vi "Lab Panel V5.20.vi"() -> ()   [LabVIEW 2013] (continued)
                      tunnel: w3938 -> [_ w3961]
                      frame #0 {
                        n2199 = case shown="True" w3955 {
                          tunnel: w3954 -> [_ w3960]
                          tunnel: w3953 -> [_ w3959]
                          tunnel: w3952 -> [_ w3958]
                          tunnel: w3951 -> [_ w3956]
                          frame False {
                          }
                          frame True {
                            n2200 = Bundle(cluster=w3956, "amps"=w3960, "volts"=w3959, "pf"=w3958) -> (w3957:cluster{"amps":dbl, "volts":dbl, "pf":dbl})
                            n2201 = local write "ON L01-2"(w3957) -> ()
                          }
                        }
                      }
                      frame #1 {
                        n2202 = Unbundle(w3965) -> ("amps"=w3964:dbl, "volts"=w3963:dbl, "pf"=w3962:dbl)
                        n2203 = case shown="True" w3966 {
                          tunnel: w3973 -> [_ w4005]
                          tunnel: w3972 -> [_ w4012]
                          tunnel: w3971 -> [_ _]
                          tunnel: w3970 -> [_ _]
                          tunnel: w3969 -> [_ w4011]
                          tunnel: w3968 -> [_ w4010]
                          tunnel: w3967 -> [_ w3975]
                          tunnel: w3964 -> [_ w4007]
                          tunnel: w3963 -> [_ w4006]
                          tunnel: w3962 -> [_ w4004]
                          tunnel: w3961 -> [_ w3996]
                          frame False {
                          }
                          frame True {
                            n2204 = local read "TDMS LAB01-2"() -> (w4009:refnum<k34>)
                            n2205 = Build Array(w4006) -> (w4001:dbl[])
                            n2206 = Build Array(w4004) -> (w4000:dbl[])
                            n2207 = Build Array(w4011) -> (w3999:dbl[])
                            n2208 = Build Array(w4012) -> (w3998:dbl[])
                            n2209 = Build Array(w4007) -> (w4003:dbl[])
                            n2210 = Build Array(w4005) -> (w4002:dbl[])
                            n2211 = Build Array(w4010) -> (w3997:dbl[])
                            n2212 = Build Array("AMPS ON", "AMPS OFF", "VOLTS", "PF", "TEMP Live", "TEMP Neut", "CYCLE") -> (w3980:string[])
                            n2213 = Bundle By Name("Y"=w4003, "t0"=w3996) -> (w3995:waveform(dbl))  [unwired: 1 in]
                            n2214 = Bundle By Name("Y"=w4002, "t0"=w3996) -> (w3994:waveform(dbl))  [unwired: 1 in]
                            n2215 = Bundle By Name("Y"=w4001, "t0"=w3996) -> (w3993:waveform(dbl))  [unwired: 1 in]
                            n2216 = Bundle By Name("Y"=w4000, "t0"=w3996) -> (w3992:waveform(dbl))  [unwired: 1 in]
                            n2217 = Bundle By Name("Y"=w3999, "t0"=w3996) -> (w3991:waveform(dbl))  [unwired: 1 in]
                            n2218 = Bundle By Name("Y"=w3998, "t0"=w3996) -> (w3990:waveform(dbl))  [unwired: 1 in]
                            n2219 = Bundle By Name("Y"=w3997, "t0"=w3996) -> (w3989:waveform(dbl))  [unwired: 1 in]
                            n2220 = Build Array(w3995, w3994, w3993, w3992, w3991, w3990, w3989) -> (w3988:waveform(dbl)[])
                            n2221 = TDMS Write(0:w4009, 5:"TEST VALUES", 7:w3980, 9:w3988) -> (4:w3979:refnum<k34>, 6:w3978:string, 15:w3977:errorcluster)  [unwired: 2 in, 1 out]
                            n2222 = TDMS Write(0:w3979, 5:w3978, 7:"TIME", 9:w3975, 11:w3977) -> (15:w3974:errorcluster)  [unwired: 1 in, 3 out]
                            n2223 = local write "data file error"(w3974) -> ()
                          }
                        }
                      }
                    }
                  }
                }
              }
              frame #2 {
                n2224 = case shown="True" w4013 {
                  tunnel: w4017 -> [_ w4022]
                  tunnel: w4016 -> [_ w4021]
                  tunnel: w4015 -> [_ w4019]
                  tunnel: w4014 -> [_ w4018]
                  frame False {
                  }
                  frame True {
                    n2225 = local read "DISP LAB02-1"() -> (w4023:T4)
                    n2226 = local read "SIG LAB02-1"() -> (w4024:T2)
                    n2227 = local read "ON L02-1"() -> (w4020:cluster{"amps":dbl, "volts":dbl, "pf":dbl})
                    n2228 = Unbundle(w4024) -> ("AMPS"=w4030:dbl, "VOLTS"=w4028:dbl, "PF"=w4027:dbl, "Tmp Live"=w4026:dbl, "Tmp Neut"=w4029:dbl)
                    n2229 = Unbundle(w4023) -> ("CYCLE"=w4025:dbl)  [unwired: 2 out]
                    n2230 = stacked-sequence {
                      tunnel: w4030 -> [w4034 w4053]
                      tunnel: w4029 -> [_ w4052]
                      tunnel: w4028 -> [w4033 w4051]
                      tunnel: w4027 -> [w4032 w4050]
                      tunnel: w4026 -> [_ w4049]
                      tunnel: w4025 -> [_ w4048]
                      tunnel: w4022 -> [_ w4047]
                      tunnel: w4021 -> [w4035 _]
                      tunnel: w4020 -> [w4031 w4045]
                      tunnel: w4019 -> [_ w4046]
                      tunnel: w4018 -> [_ w4041]
                      frame #0 {
                        n2231 = case shown="True" w4035 {
                          tunnel: w4034 -> [_ w4040]
                          tunnel: w4033 -> [_ w4039]
                          tunnel: w4032 -> [_ w4038]
                          tunnel: w4031 -> [_ w4036]
                          frame False {
                          }
                          frame True {
                            n2232 = Bundle(cluster=w4036, "amps"=w4040, "volts"=w4039, "pf"=w4038) -> (w4037:cluster{"amps":dbl, "volts":dbl, "pf":dbl})
                            n2233 = local write "ON L02-1"(w4037) -> ()
                          }
                        }
                      }
                      frame #1 {
                        n2234 = Unbundle(w4045) -> ("amps"=w4044:dbl, "volts"=w4043:dbl, "pf"=w4042:dbl)
                        n2235 = case shown="True" w4046 {
                          tunnel: w4053 -> [_ w4085]
                          tunnel: w4052 -> [_ w4092]
                          tunnel: w4051 -> [_ _]
                          tunnel: w4050 -> [_ _]
                          tunnel: w4049 -> [_ w4091]
                          tunnel: w4048 -> [_ w4090]
                          tunnel: w4047 -> [_ w4055]
                          tunnel: w4044 -> [_ w4087]
                          tunnel: w4043 -> [_ w4086]
                          tunnel: w4042 -> [_ w4084]
                          tunnel: w4041 -> [_ w4076]
                          frame False {
                          }
                          frame True {
                            n2236 = local read "TDMS LAB02-1"() -> (w4089:refnum<k34>)
                            n2237 = Build Array(w4086) -> (w4081:dbl[])
                            n2238 = Build Array(w4084) -> (w4080:dbl[])
                            n2239 = Build Array(w4091) -> (w4079:dbl[])
                            n2240 = Build Array(w4092) -> (w4078:dbl[])
                            n2241 = Build Array(w4087) -> (w4083:dbl[])
                            n2242 = Build Array(w4085) -> (w4082:dbl[])
                            n2243 = Build Array(w4090) -> (w4077:dbl[])
                            n2244 = Build Array("AMPS ON", "AMPS OFF", "VOLTS", "PF", "TEMP Live", "TEMP Neut", "CYCLE") -> (w4060:string[])
                            n2245 = Bundle By Name("Y"=w4083, "t0"=w4076) -> (w4075:waveform(dbl))  [unwired: 1 in]
                            n2246 = Bundle By Name("Y"=w4082, "t0"=w4076) -> (w4074:waveform(dbl))  [unwired: 1 in]
                            n2247 = Bundle By Name("Y"=w4081, "t0"=w4076) -> (w4073:waveform(dbl))  [unwired: 1 in]
                            n2248 = Bundle By Name("Y"=w4080, "t0"=w4076) -> (w4072:waveform(dbl))  [unwired: 1 in]
                            n2249 = Bundle By Name("Y"=w4079, "t0"=w4076) -> (w4071:waveform(dbl))  [unwired: 1 in]
                            n2250 = Bundle By Name("Y"=w4078, "t0"=w4076) -> (w4070:waveform(dbl))  [unwired: 1 in]
                            n2251 = Bundle By Name("Y"=w4077, "t0"=w4076) -> (w4069:waveform(dbl))  [unwired: 1 in]
                            n2252 = Build Array(w4075, w4074, w4073, w4072, w4071, w4070, w4069) -> (w4068:waveform(dbl)[])
                            n2253 = TDMS Write(0:w4089, 5:"TEST VALUES", 7:w4060, 9:w4068) -> (4:w4059:refnum<k34>, 6:w4058:string, 15:w4057:errorcluster)  [unwired: 2 in, 1 out]
                            n2254 = TDMS Write(0:w4059, 5:w4058, 7:"TIME", 9:w4055, 11:w4057) -> (15:w4054:errorcluster)  [unwired: 1 in, 3 out]
                            n2255 = local write "data file error"(w4054) -> ()
                          }
                        }
                      }
                    }
                  }
                }
              }
              frame #3 {
                n2256 = case shown="True" w4093 {
                  tunnel: w4097 -> [_ w4102]
                  tunnel: w4096 -> [_ w4101]
                  tunnel: w4095 -> [_ w4099]
                  tunnel: w4094 -> [_ w4098]
                  frame False {
                  }
                  frame True {
                    n2257 = local read "DISP LAB02-2"() -> (w4103:T4)
                    n2258 = local read "SIG LAB02-2"() -> (w4104:T2)
                    n2259 = local read "ON L02-2"() -> (w4100:cluster{"amps":dbl, "volts":dbl, "pf":dbl})
                    n2260 = Unbundle(w4104) -> ("AMPS"=w4110:dbl, "VOLTS"=w4108:dbl, "PF"=w4107:dbl, "Tmp Live"=w4106:dbl, "Tmp Neut"=w4109:dbl)
                    n2261 = Unbundle(w4103) -> ("CYCLE"=w4105:dbl)  [unwired: 2 out]
                    n2262 = stacked-sequence {
                      tunnel: w4110 -> [w4114 w4133]
                      tunnel: w4109 -> [_ w4132]
                      tunnel: w4108 -> [w4113 w4131]
                      tunnel: w4107 -> [w4112 w4130]
                      tunnel: w4106 -> [_ w4129]
                      tunnel: w4105 -> [_ w4128]
                      tunnel: w4102 -> [_ w4127]
                      tunnel: w4101 -> [w4115 _]
                      tunnel: w4100 -> [w4111 w4125]
                      tunnel: w4099 -> [_ w4126]
                      tunnel: w4098 -> [_ w4121]
                      frame #0 {
                        n2263 = case shown="True" w4115 {
                          tunnel: w4114 -> [_ w4120]
                          tunnel: w4113 -> [_ w4119]
                          tunnel: w4112 -> [_ w4118]
                          tunnel: w4111 -> [_ w4116]
                          frame False {
                          }
                          frame True {
                            n2264 = Bundle(cluster=w4116, "amps"=w4120, "volts"=w4119, "pf"=w4118) -> (w4117:cluster{"amps":dbl, "volts":dbl, "pf":dbl})
                            n2265 = local write "ON L02-2"(w4117) -> ()
                          }
                        }
                      }
                      frame #1 {
                        n2266 = Unbundle(w4125) -> ("amps"=w4124:dbl, "volts"=w4123:dbl, "pf"=w4122:dbl)
                        n2267 = case shown="True" w4126 {
                          tunnel: w4133 -> [_ w4165]
                          tunnel: w4132 -> [_ w4172]
                          tunnel: w4131 -> [_ _]
                          tunnel: w4130 -> [_ _]
                          tunnel: w4129 -> [_ w4171]
                          tunnel: w4128 -> [_ w4170]
                          tunnel: w4127 -> [_ w4135]
                          tunnel: w4124 -> [_ w4167]
                          tunnel: w4123 -> [_ w4166]
                          tunnel: w4122 -> [_ w4164]
                          tunnel: w4121 -> [_ w4156]
                          frame False {
                          }
                          frame True {
                            n2268 = local read "TDMS LAB02-2"() -> (w4169:refnum<k34>)
                            n2269 = Build Array(w4166) -> (w4161:dbl[])
                            n2270 = Build Array(w4164) -> (w4160:dbl[])
                            n2271 = Build Array(w4171) -> (w4159:dbl[])
                            n2272 = Build Array(w4172) -> (w4158:dbl[])
                            n2273 = Build Array(w4167) -> (w4163:dbl[])
                            n2274 = Build Array(w4165) -> (w4162:dbl[])
                            n2275 = Build Array(w4170) -> (w4157:dbl[])
                            n2276 = Build Array("AMPS ON", "AMPS OFF", "VOLTS", "PF", "TEMP Live", "TEMP Neut", "CYCLE") -> (w4140:string[])
                            n2277 = Bundle By Name("Y"=w4163, "t0"=w4156) -> (w4155:waveform(dbl))  [unwired: 1 in]
                            n2278 = Bundle By Name("Y"=w4162, "t0"=w4156) -> (w4154:waveform(dbl))  [unwired: 1 in]
                            n2279 = Bundle By Name("Y"=w4161, "t0"=w4156) -> (w4153:waveform(dbl))  [unwired: 1 in]
                            n2280 = Bundle By Name("Y"=w4160, "t0"=w4156) -> (w4152:waveform(dbl))  [unwired: 1 in]
                            n2281 = Bundle By Name("Y"=w4159, "t0"=w4156) -> (w4151:waveform(dbl))  [unwired: 1 in]
                            n2282 = Bundle By Name("Y"=w4158, "t0"=w4156) -> (w4150:waveform(dbl))  [unwired: 1 in]
                            n2283 = Bundle By Name("Y"=w4157, "t0"=w4156) -> (w4149:waveform(dbl))  [unwired: 1 in]
                            n2284 = Build Array(w4155, w4154, w4153, w4152, w4151, w4150, w4149) -> (w4148:waveform(dbl)[])
                            n2285 = TDMS Write(0:w4169, 5:"TEST VALUES", 7:w4140, 9:w4148) -> (4:w4139:refnum<k34>, 6:w4138:string, 15:w4137:errorcluster)  [unwired: 2 in, 1 out]
                            n2286 = TDMS Write(0:w4139, 5:w4138, 7:"TIME", 9:w4135, 11:w4137) -> (15:w4134:errorcluster)  [unwired: 1 in, 3 out]
                            n2287 = local write "data file error"(w4134) -> ()
                          }
                        }
                      }
                    }
                  }
                }
              }
              frame #4 {
                n2288 = case shown="True" w4173 {
                  tunnel: w4177 -> [_ w4182]
                  tunnel: w4176 -> [_ w4181]
                  tunnel: w4175 -> [_ w4179]
                  tunnel: w4174 -> [_ w4178]
                  frame False {
                  }
                  frame True {
                    n2289 = local read "DISP LAB03-1"() -> (w4183:T4)
                    n2290 = local read "SIG LAB03-1"() -> (w4184:T2)
                    n2291 = local read "ON L03-1"() -> (w4180:cluster{"amps":dbl, "volts":dbl, "pf":dbl})
                    n2292 = Unbundle(w4184) -> ("AMPS"=w4190:dbl, "VOLTS"=w4188:dbl, "PF"=w4187:dbl, "Tmp Live"=w4186:dbl, "Tmp Neut"=w4189:dbl)
                    n2293 = Unbundle(w4183) -> ("CYCLE"=w4185:dbl)  [unwired: 2 out]
                    n2294 = stacked-sequence {
                      tunnel: w4190 -> [w4194 w4213]
                      tunnel: w4189 -> [_ w4212]
                      tunnel: w4188 -> [w4193 w4211]
                      tunnel: w4187 -> [w4192 w4210]
                      tunnel: w4186 -> [_ w4209]
                      tunnel: w4185 -> [_ w4208]
                      tunnel: w4182 -> [_ w4207]
                      tunnel: w4181 -> [w4195 _]
                      tunnel: w4180 -> [w4191 w4205]
                      tunnel: w4179 -> [_ w4206]
                      tunnel: w4178 -> [_ w4201]
                      frame #0 {
                        n2295 = case shown="True" w4195 {
                          tunnel: w4194 -> [_ w4200]
                          tunnel: w4193 -> [_ w4199]
                          tunnel: w4192 -> [_ w4198]
                          tunnel: w4191 -> [_ w4196]
                          frame False {
                          }
                          frame True {
                            n2296 = Bundle(cluster=w4196, "amps"=w4200, "volts"=w4199, "pf"=w4198) -> (w4197:cluster{"amps":dbl, "volts":dbl, "pf":dbl})
                            n2297 = local write "ON L03-1"(w4197) -> ()
                          }
                        }
                      }
                      frame #1 {
                        n2298 = Unbundle(w4205) -> ("amps"=w4204:dbl, "volts"=w4203:dbl, "pf"=w4202:dbl)
                        n2299 = case shown="True" w4206 {
                          tunnel: w4213 -> [_ w4245]
                          tunnel: w4212 -> [_ w4252]
                          tunnel: w4211 -> [_ _]
                          tunnel: w4210 -> [_ _]
                          tunnel: w4209 -> [_ w4251]
                          tunnel: w4208 -> [_ w4250]
                          tunnel: w4207 -> [_ w4215]
                          tunnel: w4204 -> [_ w4247]
                          tunnel: w4203 -> [_ w4246]
                          tunnel: w4202 -> [_ w4244]
                          tunnel: w4201 -> [_ w4236]
                          frame False {
                          }
                          frame True {
                            n2300 = local read "TDMS LAB03-1"() -> (w4249:refnum<k34>)
                            n2301 = Build Array(w4246) -> (w4241:dbl[])
                            n2302 = Build Array(w4244) -> (w4240:dbl[])
                            n2303 = Build Array(w4251) -> (w4239:dbl[])
                            n2304 = Build Array(w4252) -> (w4238:dbl[])
                            n2305 = Build Array(w4247) -> (w4243:dbl[])
                            n2306 = Build Array(w4245) -> (w4242:dbl[])
                            n2307 = Build Array(w4250) -> (w4237:dbl[])
                            n2308 = Build Array("AMPS ON", "AMPS OFF", "VOLTS", "PF", "TEMP Live", "TEMP Neut", "CYCLE") -> (w4220:string[])
                            n2309 = Bundle By Name("Y"=w4243, "t0"=w4236) -> (w4235:waveform(dbl))  [unwired: 1 in]
                            n2310 = Bundle By Name("Y"=w4242, "t0"=w4236) -> (w4234:waveform(dbl))  [unwired: 1 in]
                            n2311 = Bundle By Name("Y"=w4241, "t0"=w4236) -> (w4233:waveform(dbl))  [unwired: 1 in]
                            n2312 = Bundle By Name("Y"=w4240, "t0"=w4236) -> (w4232:waveform(dbl))  [unwired: 1 in]
                            n2313 = Bundle By Name("Y"=w4239, "t0"=w4236) -> (w4231:waveform(dbl))  [unwired: 1 in]
                            n2314 = Bundle By Name("Y"=w4238, "t0"=w4236) -> (w4230:waveform(dbl))  [unwired: 1 in]
                            n2315 = Bundle By Name("Y"=w4237, "t0"=w4236) -> (w4229:waveform(dbl))  [unwired: 1 in]
                            n2316 = Build Array(w4235, w4234, w4233, w4232, w4231, w4230, w4229) -> (w4228:waveform(dbl)[])
                            n2317 = TDMS Write(0:w4249, 5:"TEST VALUES", 7:w4220, 9:w4228) -> (4:w4219:refnum<k34>, 6:w4218:string, 15:w4217:errorcluster)  [unwired: 2 in, 1 out]
                            n2318 = TDMS Write(0:w4219, 5:w4218, 7:"TIME", 9:w4215, 11:w4217) -> (15:w4214:errorcluster)  [unwired: 1 in, 3 out]
                            n2319 = local write "data file error"(w4214) -> ()
                          }
                        }
                      }
                    }
                  }
                }
              }
              frame #5 {
                n2320 = case shown="True" w4253 {
                  tunnel: w4257 -> [_ w4262]
                  tunnel: w4256 -> [_ w4261]
                  tunnel: w4255 -> [_ w4259]
                  tunnel: w4254 -> [_ w4258]
                  frame False {
                  }
                  frame True {
                    n2321 = local read "DISP LAB03-2"() -> (w4263:T4)
                    n2322 = local read "SIG LAB03-2"() -> (w4264:T2)
                    n2323 = local read "ON L03-2"() -> (w4260:cluster{"amps":dbl, "volts":dbl, "pf":dbl})
                    n2324 = Unbundle(w4264) -> ("AMPS"=w4270:dbl, "VOLTS"=w4268:dbl, "PF"=w4267:dbl, "Tmp Live"=w4266:dbl, "Tmp Neut"=w4269:dbl)
                    n2325 = Unbundle(w4263) -> ("CYCLE"=w4265:dbl)  [unwired: 2 out]
                    n2326 = stacked-sequence {
                      tunnel: w4270 -> [w4274 w4293]
                      tunnel: w4269 -> [_ w4292]
                      tunnel: w4268 -> [w4273 w4291]
                      tunnel: w4267 -> [w4272 w4290]
                      tunnel: w4266 -> [_ w4289]
                      tunnel: w4265 -> [_ w4288]
                      tunnel: w4262 -> [_ w4287]
                      tunnel: w4261 -> [w4275 _]
                      tunnel: w4260 -> [w4271 w4285]
                      tunnel: w4259 -> [_ w4286]
                      tunnel: w4258 -> [_ w4281]
                      frame #0 {
                        n2327 = case shown="True" w4275 {
                          tunnel: w4274 -> [_ w4280]
                          tunnel: w4273 -> [_ w4279]
                          tunnel: w4272 -> [_ w4278]
                          tunnel: w4271 -> [_ w4276]
                          frame False {
                          }
                          frame True {
                            n2328 = Bundle(cluster=w4276, "amps"=w4280, "volts"=w4279, "pf"=w4278) -> (w4277:cluster{"amps":dbl, "volts":dbl, "pf":dbl})
                            n2329 = local write "ON L03-2"(w4277) -> ()
                          }
                        }
                      }
                      frame #1 {
                        n2330 = Unbundle(w4285) -> ("amps"=w4284:dbl, "volts"=w4283:dbl, "pf"=w4282:dbl)
                        n2331 = case shown="True" w4286 {
                          tunnel: w4293 -> [_ w4325]
                          tunnel: w4292 -> [_ w4332]
                          tunnel: w4291 -> [_ _]
                          tunnel: w4290 -> [_ _]
                          tunnel: w4289 -> [_ w4331]
                          tunnel: w4288 -> [_ w4330]
                          tunnel: w4287 -> [_ w4295]
                          tunnel: w4284 -> [_ w4327]
                          tunnel: w4283 -> [_ w4326]
                          tunnel: w4282 -> [_ w4324]
                          tunnel: w4281 -> [_ w4316]
                          frame False {
                          }
                          frame True {
                            n2332 = local read "TDMS LAB03-2"() -> (w4329:refnum<k34>)
                            n2333 = Build Array(w4326) -> (w4321:dbl[])
                            n2334 = Build Array(w4324) -> (w4320:dbl[])
                            n2335 = Build Array(w4331) -> (w4319:dbl[])
                            n2336 = Build Array(w4332) -> (w4318:dbl[])
                            n2337 = Build Array(w4327) -> (w4323:dbl[])
                            n2338 = Build Array(w4325) -> (w4322:dbl[])
                            n2339 = Build Array(w4330) -> (w4317:dbl[])
                            n2340 = Build Array("AMPS ON", "AMPS OFF", "VOLTS", "PF", "TEMP Live", "TEMP Neut", "CYCLE") -> (w4300:string[])
                            n2341 = Bundle By Name("Y"=w4323, "t0"=w4316) -> (w4315:waveform(dbl))  [unwired: 1 in]
                            n2342 = Bundle By Name("Y"=w4322, "t0"=w4316) -> (w4314:waveform(dbl))  [unwired: 1 in]
                            n2343 = Bundle By Name("Y"=w4321, "t0"=w4316) -> (w4313:waveform(dbl))  [unwired: 1 in]
                            n2344 = Bundle By Name("Y"=w4320, "t0"=w4316) -> (w4312:waveform(dbl))  [unwired: 1 in]
                            n2345 = Bundle By Name("Y"=w4319, "t0"=w4316) -> (w4311:waveform(dbl))  [unwired: 1 in]
                            n2346 = Bundle By Name("Y"=w4318, "t0"=w4316) -> (w4310:waveform(dbl))  [unwired: 1 in]
                            n2347 = Bundle By Name("Y"=w4317, "t0"=w4316) -> (w4309:waveform(dbl))  [unwired: 1 in]
                            n2348 = Build Array(w4315, w4314, w4313, w4312, w4311, w4310, w4309) -> (w4308:waveform(dbl)[])
                            n2349 = TDMS Write(0:w4329, 5:"TEST VALUES", 7:w4300, 9:w4308) -> (4:w4299:refnum<k34>, 6:w4298:string, 15:w4297:errorcluster)  [unwired: 2 in, 1 out]
                            n2350 = TDMS Write(0:w4299, 5:w4298, 7:"TIME", 9:w4295, 11:w4297) -> (15:w4294:errorcluster)  [unwired: 1 in, 3 out]
                            n2351 = local write "data file error"(w4294) -> ()
                          }
                        }
                      }
                    }
                  }
                }
              }
              frame #6 {
                n2352 = case shown="True" w4333 {
                  tunnel: w4337 -> [_ w4342]
                  tunnel: w4336 -> [_ w4341]
                  tunnel: w4335 -> [_ w4339]
                  tunnel: w4334 -> [_ w4338]
                  frame False {
                  }
                  frame True {
                    n2353 = local read "DISP LAB04-1"() -> (w4343:T4)
                    n2354 = local read "SIG LAB04-1"() -> (w4344:T2)
                    n2355 = local read "ON L04-1"() -> (w4340:cluster{"amps":dbl, "volts":dbl, "pf":dbl})
                    n2356 = Unbundle(w4344) -> ("AMPS"=w4350:dbl, "VOLTS"=w4348:dbl, "PF"=w4347:dbl, "Tmp Live"=w4346:dbl, "Tmp Neut"=w4349:dbl)
                    n2357 = Unbundle(w4343) -> ("CYCLE"=w4345:dbl)  [unwired: 2 out]
                    n2358 = stacked-sequence {
                      tunnel: w4350 -> [w4354 w4373]
                      tunnel: w4349 -> [_ w4372]
                      tunnel: w4348 -> [w4353 w4371]
                      tunnel: w4347 -> [w4352 w4370]
                      tunnel: w4346 -> [_ w4369]
                      tunnel: w4345 -> [_ w4368]
                      tunnel: w4342 -> [_ w4367]
                      tunnel: w4341 -> [w4355 _]
                      tunnel: w4340 -> [w4351 w4365]
                      tunnel: w4339 -> [_ w4366]
                      tunnel: w4338 -> [_ w4361]
                      frame #0 {
                        n2359 = case shown="True" w4355 {
                          tunnel: w4354 -> [_ w4360]
                          tunnel: w4353 -> [_ w4359]
                          tunnel: w4352 -> [_ w4358]
                          tunnel: w4351 -> [_ w4356]
                          frame False {
                          }
                          frame True {
                            n2360 = Bundle(cluster=w4356, "amps"=w4360, "volts"=w4359, "pf"=w4358) -> (w4357:cluster{"amps":dbl, "volts":dbl, "pf":dbl})
                            n2361 = local write "ON L04-1"(w4357) -> ()
                          }
                        }
                      }
                      frame #1 {
                        n2362 = Unbundle(w4365) -> ("amps"=w4364:dbl, "volts"=w4363:dbl, "pf"=w4362:dbl)
                        n2363 = case shown="True" w4366 {
                          tunnel: w4373 -> [_ w4405]
                          tunnel: w4372 -> [_ w4412]
                          tunnel: w4371 -> [_ _]
                          tunnel: w4370 -> [_ _]
                          tunnel: w4369 -> [_ w4411]
                          tunnel: w4368 -> [_ w4410]
                          tunnel: w4367 -> [_ w4375]
                          tunnel: w4364 -> [_ w4407]
                          tunnel: w4363 -> [_ w4406]
                          tunnel: w4362 -> [_ w4404]
                          tunnel: w4361 -> [_ w4396]
                          frame False {
                          }
                          frame True {
                            n2364 = local read "TDMS LAB04-1"() -> (w4409:refnum<k34>)
                            n2365 = Build Array(w4406) -> (w4401:dbl[])
                            n2366 = Build Array(w4404) -> (w4400:dbl[])
                            n2367 = Build Array(w4411) -> (w4399:dbl[])
                            n2368 = Build Array(w4412) -> (w4398:dbl[])
                            n2369 = Build Array(w4407) -> (w4403:dbl[])
                            n2370 = Build Array(w4405) -> (w4402:dbl[])
                            n2371 = Build Array(w4410) -> (w4397:dbl[])
                            n2372 = Build Array("AMPS ON", "AMPS OFF", "VOLTS", "PF", "TEMP Live", "TEMP Neut", "CYCLE") -> (w4380:string[])
                            n2373 = Bundle By Name("Y"=w4403, "t0"=w4396) -> (w4395:waveform(dbl))  [unwired: 1 in]
                            n2374 = Bundle By Name("Y"=w4402, "t0"=w4396) -> (w4394:waveform(dbl))  [unwired: 1 in]
                            n2375 = Bundle By Name("Y"=w4401, "t0"=w4396) -> (w4393:waveform(dbl))  [unwired: 1 in]
                            n2376 = Bundle By Name("Y"=w4400, "t0"=w4396) -> (w4392:waveform(dbl))  [unwired: 1 in]
                            n2377 = Bundle By Name("Y"=w4399, "t0"=w4396) -> (w4391:waveform(dbl))  [unwired: 1 in]
                            n2378 = Bundle By Name("Y"=w4398, "t0"=w4396) -> (w4390:waveform(dbl))  [unwired: 1 in]
                            n2379 = Bundle By Name("Y"=w4397, "t0"=w4396) -> (w4389:waveform(dbl))  [unwired: 1 in]
                            n2380 = Build Array(w4395, w4394, w4393, w4392, w4391, w4390, w4389) -> (w4388:waveform(dbl)[])
                            n2381 = TDMS Write(0:w4409, 5:"TEST VALUES", 7:w4380, 9:w4388) -> (4:w4379:refnum<k34>, 6:w4378:string, 15:w4377:errorcluster)  [unwired: 2 in, 1 out]
                            n2382 = TDMS Write(0:w4379, 5:w4378, 7:"TIME", 9:w4375, 11:w4377) -> (15:w4374:errorcluster)  [unwired: 1 in, 3 out]
                            n2383 = local write "data file error"(w4374) -> ()
                          }
                        }
                      }
                    }
                  }
                }
              }
              frame #7 {
                n2384 = case shown="True" w4413 {
                  tunnel: w4417 -> [_ w4422]
                  tunnel: w4416 -> [_ w4421]
                  tunnel: w4415 -> [_ w4419]
                  tunnel: w4414 -> [_ w4418]
                  frame False {
                  }
                  frame True {
                    n2385 = local read "DISP LAB04-2"() -> (w4423:T4)
                    n2386 = local read "SIG LAB04-2"() -> (w4424:T2)
                    n2387 = local read "ON L04-2"() -> (w4420:cluster{"amps":dbl, "volts":dbl, "pf":dbl})
                    n2388 = Unbundle(w4424) -> ("AMPS"=w4430:dbl, "VOLTS"=w4428:dbl, "PF"=w4427:dbl, "Tmp Live"=w4426:dbl, "Tmp Neut"=w4429:dbl)
                    n2389 = Unbundle(w4423) -> ("CYCLE"=w4425:dbl)  [unwired: 2 out]
                    n2390 = stacked-sequence {
                      tunnel: w4430 -> [w4434 w4453]
                      tunnel: w4429 -> [_ w4452]
                      tunnel: w4428 -> [w4433 w4451]
                      tunnel: w4427 -> [w4432 w4450]
                      tunnel: w4426 -> [_ w4449]
                      tunnel: w4425 -> [_ w4448]
                      tunnel: w4422 -> [_ w4447]
                      tunnel: w4421 -> [w4435 _]
                      tunnel: w4420 -> [w4431 w4445]
                      tunnel: w4419 -> [_ w4446]
                      tunnel: w4418 -> [_ w4441]
                      frame #0 {
                        n2391 = case shown="True" w4435 {
                          tunnel: w4434 -> [_ w4440]
                          tunnel: w4433 -> [_ w4439]
                          tunnel: w4432 -> [_ w4438]
                          tunnel: w4431 -> [_ w4436]
                          frame False {
                          }
                          frame True {
                            n2392 = Bundle(cluster=w4436, "amps"=w4440, "volts"=w4439, "pf"=w4438) -> (w4437:cluster{"amps":dbl, "volts":dbl, "pf":dbl})
                            n2393 = local write "ON L04-2"(w4437) -> ()
                          }
                        }
                      }
                      frame #1 {
                        n2394 = Unbundle(w4445) -> ("amps"=w4444:dbl, "volts"=w4443:dbl, "pf"=w4442:dbl)
                        n2395 = case shown="True" w4446 {
                          tunnel: w4453 -> [_ w4485]
                          tunnel: w4452 -> [_ w4492]
                          tunnel: w4451 -> [_ _]
                          tunnel: w4450 -> [_ _]
                          tunnel: w4449 -> [_ w4491]
                          tunnel: w4448 -> [_ w4490]
                          tunnel: w4447 -> [_ w4455]
                          tunnel: w4444 -> [_ w4487]
                          tunnel: w4443 -> [_ w4486]
                          tunnel: w4442 -> [_ w4484]
                          tunnel: w4441 -> [_ w4476]
                          frame False {
                          }
                          frame True {
                            n2396 = local read "TDMS LAB04-2"() -> (w4489:refnum<k34>)
                            n2397 = Build Array(w4486) -> (w4481:dbl[])
                            n2398 = Build Array(w4484) -> (w4480:dbl[])
                            n2399 = Build Array(w4491) -> (w4479:dbl[])
                            n2400 = Build Array(w4492) -> (w4478:dbl[])
                            n2401 = Build Array(w4487) -> (w4483:dbl[])
                            n2402 = Build Array(w4485) -> (w4482:dbl[])
                            n2403 = Build Array(w4490) -> (w4477:dbl[])
                            n2404 = Build Array("AMPS ON", "AMPS OFF", "VOLTS", "PF", "TEMP Live", "TEMP Neut", "CYCLE") -> (w4460:string[])
                            n2405 = Bundle By Name("Y"=w4483, "t0"=w4476) -> (w4475:waveform(dbl))  [unwired: 1 in]
                            n2406 = Bundle By Name("Y"=w4482, "t0"=w4476) -> (w4474:waveform(dbl))  [unwired: 1 in]
                            n2407 = Bundle By Name("Y"=w4481, "t0"=w4476) -> (w4473:waveform(dbl))  [unwired: 1 in]
                            n2408 = Bundle By Name("Y"=w4480, "t0"=w4476) -> (w4472:waveform(dbl))  [unwired: 1 in]
                            n2409 = Bundle By Name("Y"=w4479, "t0"=w4476) -> (w4471:waveform(dbl))  [unwired: 1 in]
                            n2410 = Bundle By Name("Y"=w4478, "t0"=w4476) -> (w4470:waveform(dbl))  [unwired: 1 in]
                            n2411 = Bundle By Name("Y"=w4477, "t0"=w4476) -> (w4469:waveform(dbl))  [unwired: 1 in]
                            n2412 = Build Array(w4475, w4474, w4473, w4472, w4471, w4470, w4469) -> (w4468:waveform(dbl)[])
                            n2413 = TDMS Write(0:w4489, 5:"TEST VALUES", 7:w4460, 9:w4468) -> (4:w4459:refnum<k34>, 6:w4458:string, 15:w4457:errorcluster)  [unwired: 2 in, 1 out]
                            n2414 = TDMS Write(0:w4459, 5:w4458, 7:"TIME", 9:w4455, 11:w4457) -> (15:w4454:errorcluster)  [unwired: 1 in, 3 out]
                            n2415 = local write "data file error"(w4454) -> ()
                          }
                        }
                      }
                    }
                  }
                }
              }
              frame #8 {
                n2416 = case shown="True" w4493 {
                  tunnel: w4497 -> [_ w4502]
                  tunnel: w4496 -> [_ w4501]
                  tunnel: w4495 -> [_ w4499]
                  tunnel: w4494 -> [_ w4498]
                  frame False {
                  }
                  frame True {
                    n2417 = local read "DISP LAB05-1"() -> (w4503:T4)
                    n2418 = local read "SIG LAB05-1"() -> (w4504:T2)
                    n2419 = local read "ON L05-1"() -> (w4500:cluster{"amps":dbl, "volts":dbl, "pf":dbl})
                    n2420 = Unbundle(w4504) -> ("AMPS"=w4510:dbl, "VOLTS"=w4508:dbl, "PF"=w4507:dbl, "Tmp Live"=w4506:dbl, "Tmp Neut"=w4509:dbl)
                    n2421 = Unbundle(w4503) -> ("CYCLE"=w4505:dbl)  [unwired: 2 out]
                    n2422 = stacked-sequence {
                      tunnel: w4510 -> [w4514 w4533]
                      tunnel: w4509 -> [_ w4532]
                      tunnel: w4508 -> [w4513 w4531]
                      tunnel: w4507 -> [w4512 w4530]
                      tunnel: w4506 -> [_ w4529]
                      tunnel: w4505 -> [_ w4528]
                      tunnel: w4502 -> [_ w4527]
                      tunnel: w4501 -> [w4515 _]
                      tunnel: w4500 -> [w4511 w4525]
                      tunnel: w4499 -> [_ w4526]
                      tunnel: w4498 -> [_ w4521]
                      frame #0 {
                        n2423 = case shown="True" w4515 {
                          tunnel: w4514 -> [_ w4520]
                          tunnel: w4513 -> [_ w4519]
                          tunnel: w4512 -> [_ w4518]
                          tunnel: w4511 -> [_ w4516]
                          frame False {
                          }
                          frame True {
                            n2424 = Bundle(cluster=w4516, "amps"=w4520, "volts"=w4519, "pf"=w4518) -> (w4517:cluster{"amps":dbl, "volts":dbl, "pf":dbl})
                            n2425 = local write "ON L05-1"(w4517) -> ()
                          }
                        }
                      }
                      frame #1 {
                        n2426 = Unbundle(w4525) -> ("amps"=w4524:dbl, "volts"=w4523:dbl, "pf"=w4522:dbl)
                        n2427 = case shown="True" w4526 {
                          tunnel: w4533 -> [_ w4565]
                          tunnel: w4532 -> [_ w4572]
                          tunnel: w4531 -> [_ _]
                          tunnel: w4530 -> [_ _]
                          tunnel: w4529 -> [_ w4571]
                          tunnel: w4528 -> [_ w4570]
                          tunnel: w4527 -> [_ w4535]
                          tunnel: w4524 -> [_ w4567]
                          tunnel: w4523 -> [_ w4566]
                          tunnel: w4522 -> [_ w4564]
                          tunnel: w4521 -> [_ w4556]
                          frame False {
                          }
                          frame True {
                            n2428 = local read "TDMS LAB05-1"() -> (w4569:refnum<k34>)
                            n2429 = Build Array(w4566) -> (w4561:dbl[])
                            n2430 = Build Array(w4564) -> (w4560:dbl[])
                            n2431 = Build Array(w4571) -> (w4559:dbl[])
                            n2432 = Build Array(w4572) -> (w4558:dbl[])
                            n2433 = Build Array(w4567) -> (w4563:dbl[])
                            n2434 = Build Array(w4565) -> (w4562:dbl[])
                            n2435 = Build Array(w4570) -> (w4557:dbl[])
                            n2436 = Build Array("AMPS ON", "AMPS OFF", "VOLTS", "PF", "TEMP Live", "TEMP Neut", "CYCLE") -> (w4540:string[])
                            n2437 = Bundle By Name("Y"=w4563, "t0"=w4556) -> (w4555:waveform(dbl))  [unwired: 1 in]
                            n2438 = Bundle By Name("Y"=w4562, "t0"=w4556) -> (w4554:waveform(dbl))  [unwired: 1 in]
                            n2439 = Bundle By Name("Y"=w4561, "t0"=w4556) -> (w4553:waveform(dbl))  [unwired: 1 in]
                            n2440 = Bundle By Name("Y"=w4560, "t0"=w4556) -> (w4552:waveform(dbl))  [unwired: 1 in]
                            n2441 = Bundle By Name("Y"=w4559, "t0"=w4556) -> (w4551:waveform(dbl))  [unwired: 1 in]
                            n2442 = Bundle By Name("Y"=w4558, "t0"=w4556) -> (w4550:waveform(dbl))  [unwired: 1 in]
                            n2443 = Bundle By Name("Y"=w4557, "t0"=w4556) -> (w4549:waveform(dbl))  [unwired: 1 in]
                            n2444 = Build Array(w4555, w4554, w4553, w4552, w4551, w4550, w4549) -> (w4548:waveform(dbl)[])
                            n2445 = TDMS Write(0:w4569, 5:"TEST VALUES", 7:w4540, 9:w4548) -> (4:w4539:refnum<k34>, 6:w4538:string, 15:w4537:errorcluster)  [unwired: 2 in, 1 out]
                            n2446 = TDMS Write(0:w4539, 5:w4538, 7:"TIME", 9:w4535, 11:w4537) -> (15:w4534:errorcluster)  [unwired: 1 in, 3 out]
                            n2447 = local write "data file error"(w4534) -> ()
                          }
                        }
                      }
                    }
                  }
                }
              }
              frame #9 {
                n2448 = case shown="True" w4573 {
                  tunnel: w4577 -> [_ w4582]
                  tunnel: w4576 -> [_ w4581]
                  tunnel: w4575 -> [_ w4579]
                  tunnel: w4574 -> [_ w4578]
                  frame False {
                  }
                  frame True {
                    n2449 = local read "DISP LAB05-2"() -> (w4583:T4)
                    n2450 = local read "SIG LAB05-2"() -> (w4584:T2)
                    n2451 = local read "ON L05-2"() -> (w4580:cluster{"amps":dbl, "volts":dbl, "pf":dbl})
                    n2452 = Unbundle(w4584) -> ("AMPS"=w4590:dbl, "VOLTS"=w4588:dbl, "PF"=w4587:dbl, "Tmp Live"=w4586:dbl, "Tmp Neut"=w4589:dbl)
                    n2453 = Unbundle(w4583) -> ("CYCLE"=w4585:dbl)  [unwired: 2 out]
                    n2454 = stacked-sequence {
                      tunnel: w4590 -> [w4594 w4613]
                      tunnel: w4589 -> [_ w4612]
                      tunnel: w4588 -> [w4593 w4611]
                      tunnel: w4587 -> [w4592 w4610]
                      tunnel: w4586 -> [_ w4609]
                      tunnel: w4585 -> [_ w4608]
                      tunnel: w4582 -> [_ w4607]
                      tunnel: w4581 -> [w4595 _]
                      tunnel: w4580 -> [w4591 w4605]
                      tunnel: w4579 -> [_ w4606]
                      tunnel: w4578 -> [_ w4601]
                      frame #0 {
                        n2455 = case shown="True" w4595 {
                          tunnel: w4594 -> [_ w4600]
                          tunnel: w4593 -> [_ w4599]
                          tunnel: w4592 -> [_ w4598]
                          tunnel: w4591 -> [_ w4596]
                          frame False {
                          }
                          frame True {
                            n2456 = Bundle(cluster=w4596, "amps"=w4600, "volts"=w4599, "pf"=w4598) -> (w4597:cluster{"amps":dbl, "volts":dbl, "pf":dbl})
                            n2457 = local write "ON L05-2"(w4597) -> ()
                          }
                        }
                      }
                      frame #1 {
                        n2458 = Unbundle(w4605) -> ("amps"=w4604:dbl, "volts"=w4603:dbl, "pf"=w4602:dbl)
                        n2459 = case shown="True" w4606 {
                          tunnel: w4613 -> [_ w4645]
                          tunnel: w4612 -> [_ w4652]
                          tunnel: w4611 -> [_ _]
                          tunnel: w4610 -> [_ _]
                          tunnel: w4609 -> [_ w4651]
                          tunnel: w4608 -> [_ w4650]
                          tunnel: w4607 -> [_ w4615]
                          tunnel: w4604 -> [_ w4647]
                          tunnel: w4603 -> [_ w4646]
                          tunnel: w4602 -> [_ w4644]
                          tunnel: w4601 -> [_ w4636]
                          frame False {
                          }
                          frame True {
                            n2460 = local read "TDMS LAB05-2"() -> (w4649:refnum<k34>)
                            n2461 = Build Array(w4646) -> (w4641:dbl[])
                            n2462 = Build Array(w4644) -> (w4640:dbl[])
                            n2463 = Build Array(w4651) -> (w4639:dbl[])
                            n2464 = Build Array(w4652) -> (w4638:dbl[])
                            n2465 = Build Array(w4647) -> (w4643:dbl[])
                            n2466 = Build Array(w4645) -> (w4642:dbl[])
                            n2467 = Build Array(w4650) -> (w4637:dbl[])
                            n2468 = Build Array("AMPS ON", "AMPS OFF", "VOLTS", "PF", "TEMP Live", "TEMP Neut", "CYCLE") -> (w4620:string[])
                            n2469 = Bundle By Name("Y"=w4643, "t0"=w4636) -> (w4635:waveform(dbl))  [unwired: 1 in]
                            n2470 = Bundle By Name("Y"=w4642, "t0"=w4636) -> (w4634:waveform(dbl))  [unwired: 1 in]
                            n2471 = Bundle By Name("Y"=w4641, "t0"=w4636) -> (w4633:waveform(dbl))  [unwired: 1 in]
                            n2472 = Bundle By Name("Y"=w4640, "t0"=w4636) -> (w4632:waveform(dbl))  [unwired: 1 in]
                            n2473 = Bundle By Name("Y"=w4639, "t0"=w4636) -> (w4631:waveform(dbl))  [unwired: 1 in]
                            n2474 = Bundle By Name("Y"=w4638, "t0"=w4636) -> (w4630:waveform(dbl))  [unwired: 1 in]
                            n2475 = Bundle By Name("Y"=w4637, "t0"=w4636) -> (w4629:waveform(dbl))  [unwired: 1 in]
                            n2476 = Build Array(w4635, w4634, w4633, w4632, w4631, w4630, w4629) -> (w4628:waveform(dbl)[])
                            n2477 = TDMS Write(0:w4649, 5:"TEST VALUES", 7:w4620, 9:w4628) -> (4:w4619:refnum<k34>, 6:w4618:string, 15:w4617:errorcluster)  [unwired: 2 in, 1 out]
                            n2478 = TDMS Write(0:w4619, 5:w4618, 7:"TIME", 9:w4615, 11:w4617) -> (15:w4614:errorcluster)  [unwired: 1 in, 3 out]
                            n2479 = local write "data file error"(w4614) -> ()
                          }
                        }
                      }
                    }
                  }
                }
              }
            }
          }
          frame #13 {
            # "display test values on chart"
            n2480 = local read "jig cycle"() -> (w4657:dbl)
            n2481 = local read "on loops"() -> (w4659:dbl)
            n2482 = Add(x=w4659, y=2) -> (x+y=w4656:dbl)
            n2483 = Equal?(x=w4657, y=1) -> (x = y?=w4655:bool)
            n2484 = Equal?(x=w4657, y=w4656) -> (x = y?=w4654:bool)
            n2485 = Or(x=w4655, y=w4654) -> (x .or. y?=w4653:bool)
            "graph flag" <- w4653
            n2486 = global write "Global display 3.vi" "graph flag"(w4653) -> ()
            n2487 = case shown="True" w4653 {
              frame False {
              }
              frame True {
                n2488 = local read "SIG LAB05-1"() -> (w4702:T2)
                n2489 = local read "SIG LAB04-2"() -> (w4703:T2)
                n2490 = local read "SIG LAB05-2"() -> (w4701:T2)
                n2491 = local read "SIG LAB04-1"() -> (w4704:T2)
                n2492 = local read "SIG LAB03-1"() -> (w4706:T2)
                n2493 = local read "SIG LAB03-2"() -> (w4705:T2)
                n2494 = local read "SIG LAB01-1"() -> (w4710:T2)
                n2495 = local read "SIG LAB02-2"() -> (w4707:T2)
                n2496 = local read "SIG LAB02-1"() -> (w4708:T2)
                n2497 = local read "SIG LAB01-2"() -> (w4709:T2)
                n2498 = Unbundle(w4703) -> ("AMPS"=w4693:dbl, "VOLTS"=w4683:dbl, "Tmp Live"=w4673:dbl, "Tmp Neut"=w4663:dbl)  [unwired: 1 out]
                n2499 = Unbundle(w4702) -> ("AMPS"=w4692:dbl, "VOLTS"=w4682:dbl, "Tmp Live"=w4672:dbl, "Tmp Neut"=w4662:dbl)  [unwired: 1 out]
                n2500 = Unbundle(w4701) -> ("AMPS"=w4691:dbl, "VOLTS"=w4681:dbl, "Tmp Live"=w4671:dbl, "Tmp Neut"=w4661:dbl)  [unwired: 1 out]
                n2501 = Unbundle(w4704) -> ("AMPS"=w4694:dbl, "VOLTS"=w4684:dbl, "Tmp Live"=w4674:dbl, "Tmp Neut"=w4664:dbl)  [unwired: 1 out]
                n2502 = Unbundle(w4705) -> ("AMPS"=w4695:dbl, "VOLTS"=w4685:dbl, "Tmp Live"=w4675:dbl, "Tmp Neut"=w4665:dbl)  [unwired: 1 out]
                n2503 = Unbundle(w4706) -> ("AMPS"=w4696:dbl, "VOLTS"=w4686:dbl, "Tmp Live"=w4676:dbl, "Tmp Neut"=w4666:dbl)  [unwired: 1 out]
                n2504 = Unbundle(w4707) -> ("AMPS"=w4697:dbl, "VOLTS"=w4687:dbl, "Tmp Live"=w4677:dbl, "Tmp Neut"=w4667:dbl)  [unwired: 1 out]
                n2505 = Unbundle(w4708) -> ("AMPS"=w4698:dbl, "VOLTS"=w4688:dbl, "Tmp Live"=w4678:dbl, "Tmp Neut"=w4668:dbl)  [unwired: 1 out]
                n2506 = Unbundle(w4710) -> ("AMPS"=w4700:dbl, "VOLTS"=w4690:dbl, "Tmp Live"=w4680:dbl, "Tmp Neut"=w4670:dbl)  [unwired: 1 out]
                n2507 = Unbundle(w4709) -> ("AMPS"=w4699:dbl, "VOLTS"=w4689:dbl, "Tmp Live"=w4679:dbl, "Tmp Neut"=w4669:dbl)  [unwired: 1 out]
                n2508 = stacked-sequence {
                  tunnel: w4700 -> [w4742 _ _]
                  tunnel: w4699 -> [w4741 _ _]
                  tunnel: w4698 -> [w4732 _ _]
                  tunnel: w4697 -> [w4731 _ _]
                  tunnel: w4696 -> [w4721 _ _]
                  tunnel: w4695 -> [w4720 _ _]
                  tunnel: w4694 -> [_ w4765 _]
                  tunnel: w4693 -> [_ w4764 _]
                  tunnel: w4692 -> [_ w4754 _]
                  tunnel: w4691 -> [_ w4753 _]
                  tunnel: w4690 -> [w4739 _ _]
                  tunnel: w4689 -> [w4738 _ _]
                  tunnel: w4688 -> [w4729 _ _]
                  tunnel: w4687 -> [w4728 _ _]
                  tunnel: w4686 -> [w4719 _ _]
                  tunnel: w4685 -> [w4718 _ _]
                  tunnel: w4684 -> [_ w4763 _]
                  tunnel: w4683 -> [_ w4762 _]
                  tunnel: w4682 -> [_ w4752 _]
                  tunnel: w4681 -> [_ w4751 _]
                  tunnel: w4680 -> [w4736 _ _]
                  tunnel: w4679 -> [w4734 _ _]
                  tunnel: w4678 -> [w4725 _ _]
                  tunnel: w4677 -> [w4723 _ _]
                  tunnel: w4676 -> [w4717 _ _]
                  tunnel: w4675 -> [w4715 _ _]
                  tunnel: w4674 -> [_ w4761 _]
                  tunnel: w4673 -> [_ w4759 _]
                  tunnel: w4672 -> [_ w4750 _]
                  tunnel: w4671 -> [_ w4748 _]
